vi "Triangle-NodeBox containment test.vi"(1 "NodeBox":T2={"Face 0"={"V0"=[], "V1"=[], "V2"=[], "V3"=[], "E0"=[], "E1"=[], "E2"=[], "E3"=[], "n^"=[], "nE0^"=[], "nE1^"=[], "nE2^"=[], "nE3^"=[]}, "Face 1"={"V0"=[], "V1"=[], "V2"=[], "V3"=[], "E0"=[], "E1"=[], "E2"=[], "E3"=[], "n^"=[], "nE0^"=[], "nE1^"=[], "nE2^"=[], "nE3^"=[]}, "Face 2"={"V0"=[], "V1"=[], "V2"=[], "V3"=[], "E0"=[], "E1"=[], "E2"=[], "E3"=[], "n^"=[], "nE0^"=[], "nE1^"=[], "nE2^"=[], "nE3^"=[]}, "Face 3"={"V0"=[], "V1"=[], "V2"=[], "V3"=[], "E0"=[], "E1"=[], "E2"=[], "E3"=[], "n^"=[], "nE0^"=[], "nE1^"=[], "nE2^"=[], "nE3^"=[]}, "Face 4"={"V0"=[], "V1"=[], "V2"=[], "V3"=[], "E0"=[], "E1"=[], "E2"=[], "E3"=[], "n^"=[], "nE0^"=[], "nE1^"=[], "nE2^"=[], "nE3^"=[]}, "Face 5"={"V0"=[], "V1"=[], "V2"=[], "V3"=[], "E0"=[], "E1"=[], "E2"=[], "E3"=[], "n^"=[], "nE0^"=[], "nE1^"=[], "nE2^"=[], "nE3^"=[]}, "Level"=-1, "Pmax"=[], "Pmin"=[], "Parent"=-1, "Child 1"=-1, "Child 2"=-1, "Child 3"=-1, "Child 4"=-1, "Child 5"=-1, "Child 6"=-1, "Child 7"=-1, "Child 8"=-1, "Triangles"=[], "is leaf node"=FALSE}, 2 "Triangle":T1) -> (0 "Triangle is in NodeBox":bool)   [LabVIEW 2014]
uses:
  Typedefs/TreeNodeBox.ctl
  Typedefs/Quad.ctl
  Typedefs/Triangle.ctl
panel:
  # "PN 17/01/2015"
  # "Vertices"
  # "Edges"
  # "Unit normal"
  # "pre-store"
  # "Vertices"
  # "Edges"
  # "Unit normal"
  # "Edge unit normals"
  # "Vertices"
  # "Edges"
  # "Unit normal"
  # "Edge unit normals"
  # "Vertices"
  # "Edges"
  # "Unit normal"
  # "Edge unit normals"
  # "Vertices"
  # "Edges"
  # "Unit normal"
  # "Edge unit normals"
  # "Vertices"
  # "Edges"
  # "Unit normal"
  # "Edge unit normals"
  # "Vertices"
  # "Edges"
  # "Unit normal"
  # "Edge unit normals"
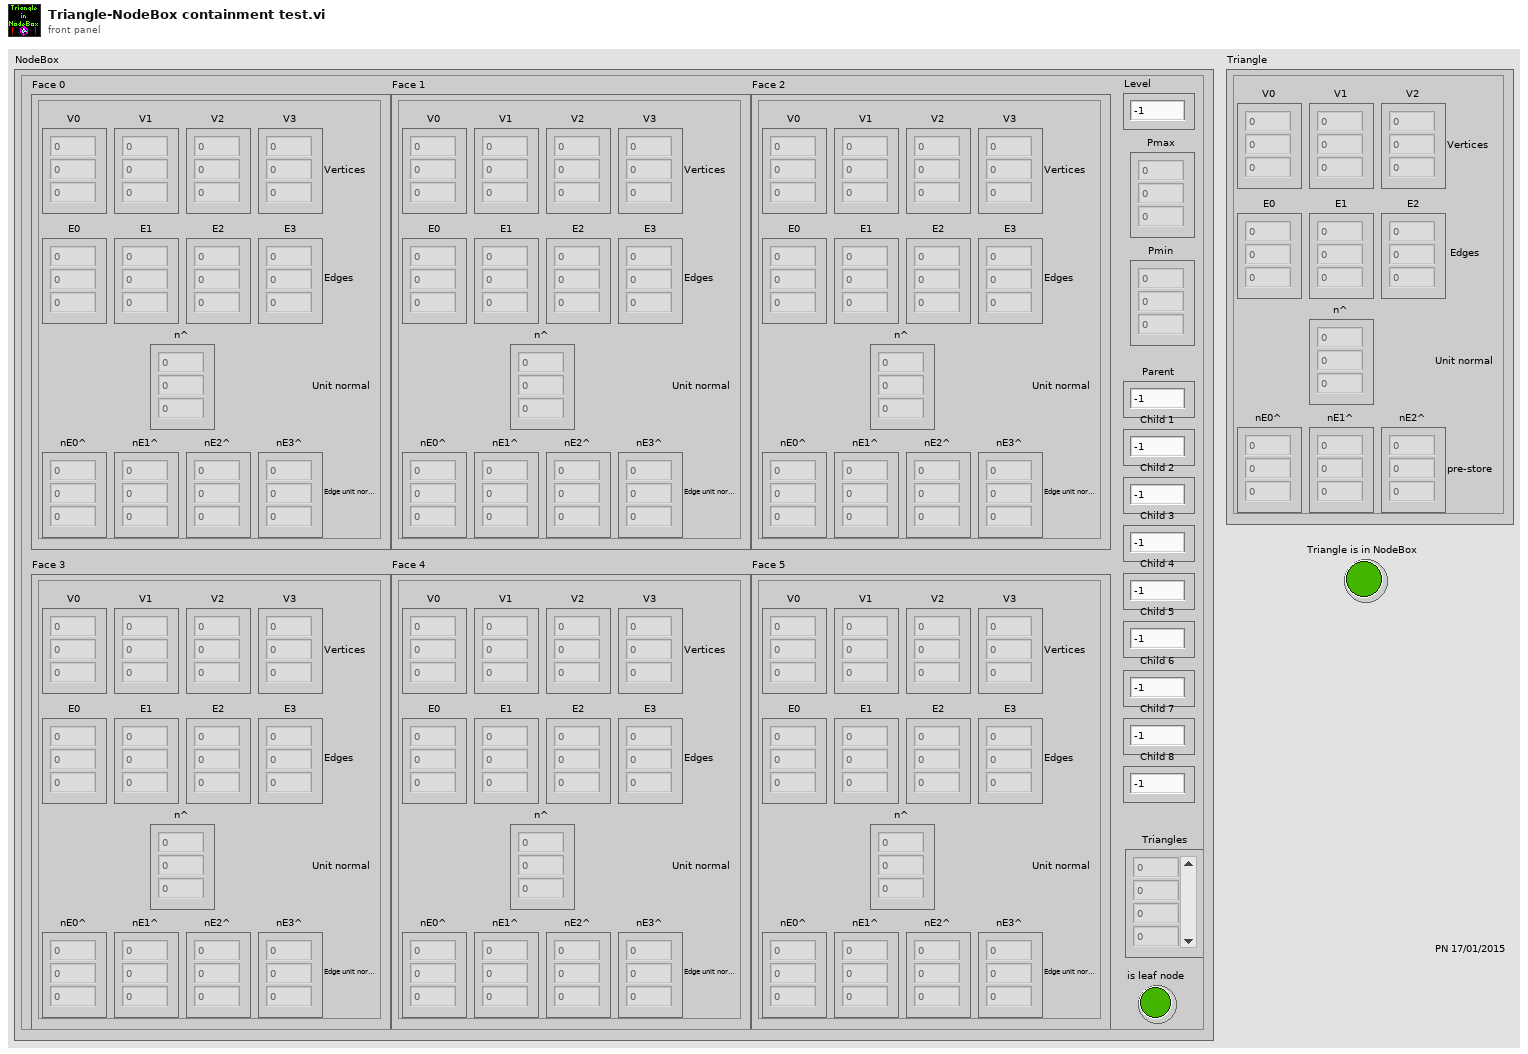
[diagram p1: front panel]
types:
  T1 = typedef "Triangle.ctl" = cluster{"V0":sgl[], "V1":sgl[], "V2":sgl[], "E0":sgl[], "E1":sgl[], "E2":sgl[], "n^":sgl[], "nE0^":sgl[], "nE1^":sgl[], "nE2^":sgl[]}
  T2 = typedef "TreeNodeBox.ctl" = cluster{"Face 0":T3, "Face 1":T3, "Face 2":T3, "Face 3":T3, "Face 4":T3, "Face 5":T3, "Level":i32, "Pmax":sgl[], "Pmin":sgl[], "Parent":i32, "Child 1":i32, "Child 2":i32, "Child 3":i32, "Child 4":i32, "Child 5":i32, "Child 6":i32, "Child 7":i32, "Child 8":i32, "Triangles":i32[], "is leaf node":bool}
  T3 = typedef "Quad.ctl" = cluster{"V0":sgl[], "V1":sgl[], "V2":sgl[], "V3":sgl[], "E0":sgl[], "E1":sgl[], "E2":sgl[], "E3":sgl[], "n^":sgl[], "nE0^":sgl[], "nE1^":sgl[], "nE2^":sgl[], "nE3^":sgl[]}
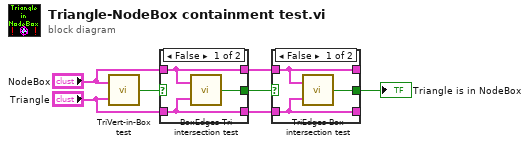
[diagram p0: block diagram]
diagram:
  n1 = call "TriVert-in-Box test.vi"("Triangle"="Triangle", "Box"="NodeBox") -> ("Vertex is inside box"=w7:bool)
  n2 = case shown="False" w7 {
    selector: w7 -> [_ w11]
    tunnel: "NodeBox" -> [w10 w13]
    tunnel: "Triangle" -> [w9 w12]
    tunnel: [w10 w13] -> w3
    tunnel: [w9 w12] -> w2
    tunnel: [w8 w11] -> w4
    frame False {
      n3 = call "BoxEdges-Tri intersection test.vi"("Triangle"=w9, "Box"=w10) -> ("Intersection"=w8:bool)
    }
    frame True {
    }
  }
  n4 = case shown="False" w4 {
    selector: w4 -> [_ w17]
    tunnel: w3 -> [w15 w19]
    tunnel: w2 -> [w14 w18]
    tunnel: [w15 w19] -> _
    tunnel: [w14 w18] -> _
    tunnel: [w16 w17] -> w1
    frame False {
      n5 = call "TriEdges-Box intersection test.vi"("Triangle"=w14, "Box"=w15) -> ("Intersection"=w16:bool)
    }
    frame True {
    }
  }
  "Triangle is in NodeBox" <- w1
